vi "Genelogy.vi"(8 "error in":errorcluster, 10 "PNSN Regex":string="^(P:)(\\w{2}-\\w{6})(R:)(\\w{2})(S:)((\\w{3})(\\d{2})(\\d{2})(\\d{5}))$", 11 "Barcode":string="P:10-000001R:04S:QMC2200123") -> (0 "error out":errorcluster, 1 "SerialNumber":string, 2 "PartNumber":string, 3 "Revision":string)   [LabVIEW 2021, in "PreUUT.lvclass"]
uses:
  PreUUT.lvclass
  <vilib>/regexp/Match Regular Expression.xnode
panel:
  out "PN_SN":string
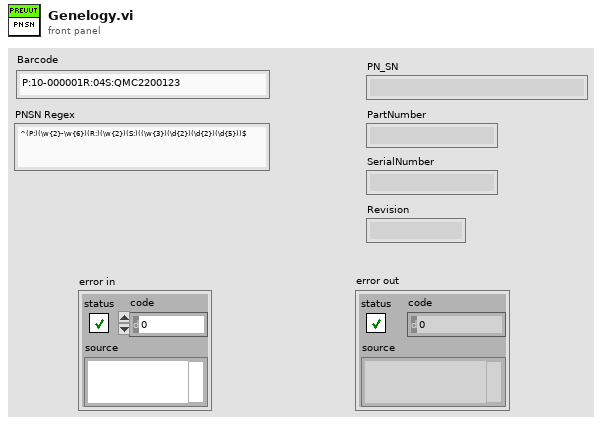
[diagram p1: front panel]
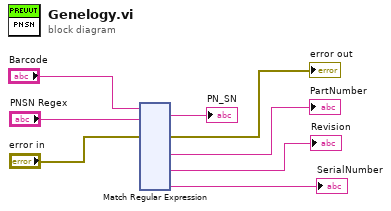
[diagram p0: block diagram]
diagram:
  n1 = xnode "Match Regular Expression"("input string"="Barcode", "regular expression"="PNSN Regex", "error in"="error in") -> ("whole match"=→"PN_SN":string, "error out"=→"error out":errorcluster, "submatch 2"=→"PartNumber":string, "submatch 4"=→"Revision":string, "submatch 6"=→"SerialNumber":string)  [unwired: 3 in, 6 out]
